vi "get_rawData.vi"(8 "error in (no error)":errorcluster, 11 "HGF_NetworkData":refnum<class "HGF_NetworkVisitor.lvclass">) -> (0 "error out":errorcluster, 2 "rawData":variant, 3 "dup HGF_NetworkData":refnum<class "HGF_NetworkVisitor.lvclass">)   [LabVIEW 2014, in "HGF_BaseClasses.lvlib" / "HGF_NetworkVisitor.lvclass"]
uses:
  HGF_NetworkVisitor.lvclass
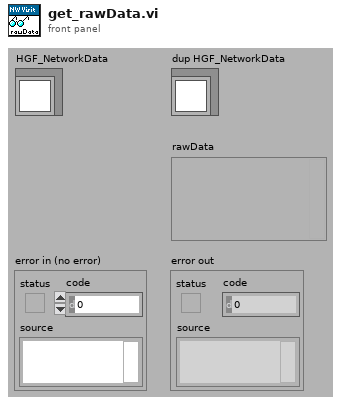
[diagram p1: front panel]
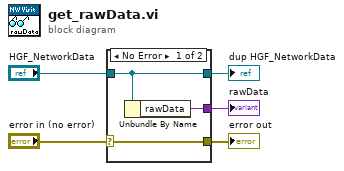
[diagram p0: block diagram]
diagram:
  n1 = case shown="No Error" "error in (no error)" {
    selector: "error in (no error)" -> [w8 w9]
    tunnel: [w8 w9] -> w4
    tunnel: [w7 w10] -> w2
    tunnel: "HGF_NetworkData" -> [w7 w10]
    tunnel: [w6 _] -> w1
    frame No Error {
      n2 = Unbundle By Name(w7) -> ("rawData"=w6:variant)
    }
    frame Error {
    }
  }
  "error out" <- w4
  "dup HGF_NetworkData" <- w2
  "rawData" <- w1
